vi "Enable or Disable Button.vi"(8 "Error In":errorcluster, 9 "Mark Selected Errors As Read Button Reference":refnum<vi>, 10 "MCL NewVal":i32[](array[numeric]), 11 "Handled Errors (MCL Display Order)":T1[](array[typedef])) -> (0 "Error Out":errorcluster)   [LabVIEW 2023, in "Error Manager.lvlib" / "Mark Selected Errors As Read Button.lvclass"]
doc: "This VI determines whether the \"Mark Selected Errors As Read\" button should be enabled or disabled and greyed out. The button should be enabled only when the user has selected one or more rows that represent unread errors.\n\nThis VI also controls the Boolean Text of the button. If 0 or 1 MCL rows are selected, the boolean text is set to \"Mark Selected Error As Read\". If two or more rows are selected, the boolean text is set to \"Mark Selected Errors As Read\"."
uses:
  Mark Selected Errors As Read Button.lvclass
  Mark Selected Errors As Read Button.lvclass/Mark Selected Errors As Read Button.ctl
  Private VIs/Read-Unread Status (enum).ctl
  Error Manager.lvlib
  Private VIs/Handled Error (cluster).ctl
panel:
  out "Number of MCL rows selected":i32
  # "Development\nControls or indicators that are useful for development or testing, but which are not outputs of the VI."
  # "Input\nInputs to the VI"
  # "Output\nOutputs of the VI"
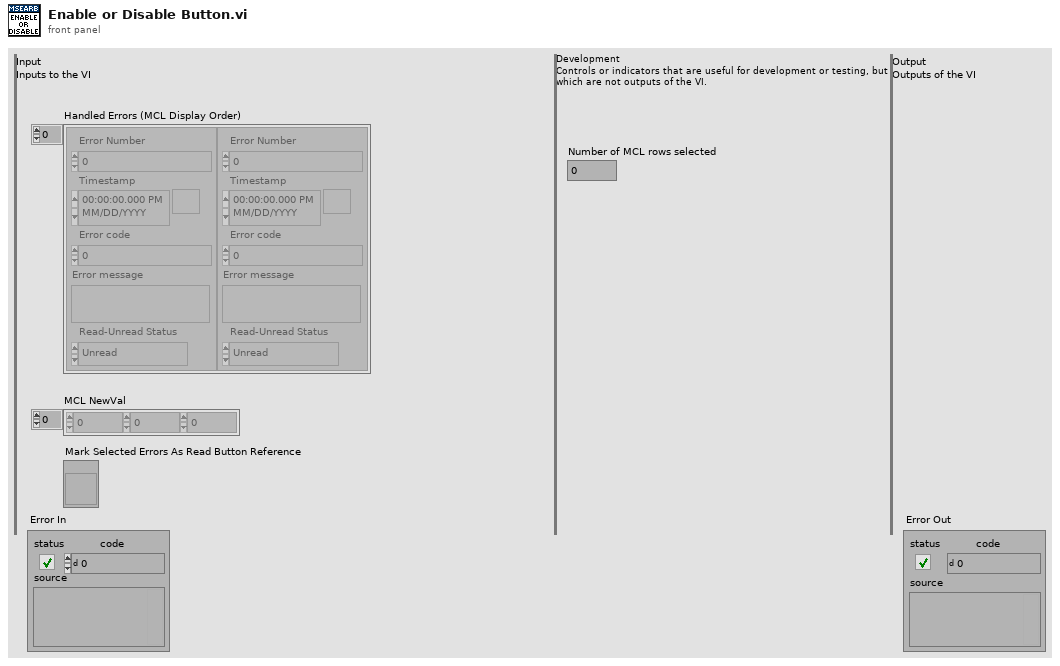
[diagram p1: front panel]
types:
  T1 = typedef "Error Manager.lvlib/Handled Error (cluster).ctl" = cluster{"Error Number":i32, "Timestamp":timestamp, "Error code":i32, "Error message":string, "Read-Unread Status":T2}
  T2 = typedef "Error Manager.lvlib/Read-Unread Status (enum).ctl" = enum16{"Unread", "Read"}
  T3 = enum8{"Enabled", "Disabled", "Disabled and Grayed Out"}
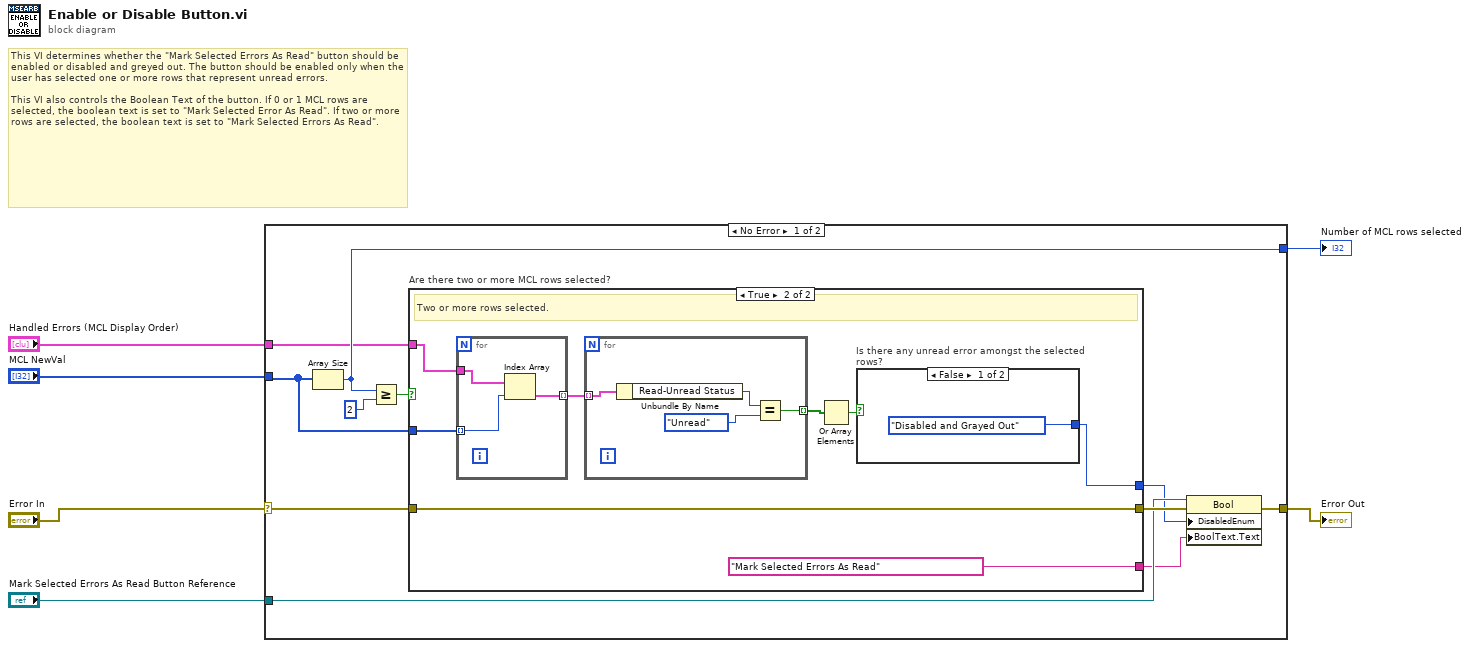
[diagram p0: block diagram]
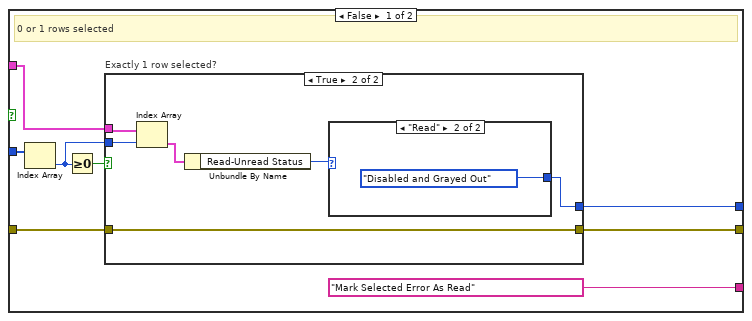
[diagram p2: hidden frame]
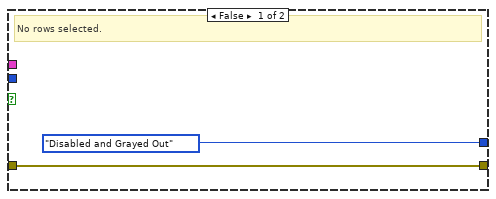
[diagram p3: hidden frame]
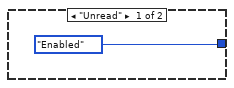
[diagram p4: hidden frame]
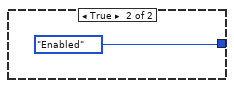
[diagram p5: hidden frame]
diagram:
  # "This VI determines whether the \"Mark Selected Errors As Read\" button should be enabled or disabled and greyed out. The button should be enabled only when the user has selected one or more rows that represent unread errors.\n\nThis VI also controls the Boolean Text of the button. If 0 or 1 MCL rows are selected, the boolean text is set to \"Mark Selected Error As Read\". If two or more rows are selected, the boolean text is set to \"Mark Selected Errors As Read\"."
  n1 = case shown="No Error" "Error In" {
    selector: "Error In" -> [w17 w53]
    tunnel: [w11 w53] -> w5
    tunnel: "Handled Errors (MCL Display Order)" -> [w8 _]
    tunnel: "MCL NewVal" -> [w12 _]
    tunnel: [w13 _] -> w2
    tunnel: "Mark Selected Errors As Read Button Reference" -> [w10 _]
    frame No Error {
      n2 = Array Size(array=w12) -> (size(s)=w13:i32)
      n3 = Greater Or Equal?(x=w13, y=2) -> (x >= y?=w14:bool)
      n4 = case "Are there two or more MCL rows selected?" shown="True" w14 {
        tunnel: w17 -> [w25 w43]
        tunnel: [w23 w43] -> w15
        tunnel: w12 -> [w24 w40]
        tunnel: [w21 w36] -> w9
        tunnel: w8 -> [w20 w41]
        tunnel: ["Mark Selected Error As Read" ("Boolean Text.Text") "Mark Selected Errors As Read" ("Boolean Text.Text")] -> w7
        frame False {
          # "0 or 1 rows selected"
          n5 = Index Array(array=w24) -> (element=w19:i32)  [unwired: 1 in]
          n6 = Greater Or Equal To 0?(x=w19) -> (x >= 0?=w22:bool)
          n7 = case "Exactly 1 row selected?" shown="True" w22 {
            tunnel: w25 -> [w27 w33]
            tunnel: [w27 w33] -> w23
            tunnel: [T3."Disabled and Grayed Out" ("Disabled") w28] -> w21
            tunnel: w20 -> [_ w31]
            tunnel: w19 -> [_ w32]
            frame False {
              # "No rows selected."
            }
            frame True {
              n8 = Index Array(array=w31, index=w32) -> (element=w30:T1)
              n9 = Unbundle By Name(w30) -> ("Read-Unread Status"=w29:T2)
              n10 = case shown="\"Read\"" w29 {
                tunnel: [T3."Enabled" ("Disabled") T3."Disabled and Grayed Out" ("Disabled")] -> w28
                frame "Unread" {
                }
                frame "Read" {
                }
              }
            }
          }
        }
        frame True {
          # "Two or more rows selected."
          n11 = for {
            tunnel: w41 -> [w52]
            tunnel: w40 -> [w51] mode=indexing
            tunnel: [w50] -> w39 mode=indexing
            n12 = Index Array(array=w52, index=w51) -> (element=w50:T1)
          }
          n13 = for {
            tunnel: w39 -> [w49] mode=indexing
            tunnel: [w46] -> w38 mode=indexing
            n14 = Unbundle By Name(w49) -> ("Read-Unread Status"=w48:T2)
            n15 = Equal?(x=w48, y=Read-Unread_Status_(enum)."Unread") -> (x = y?=w46:bool)
          }
          n16 = Or Array Elements(Boolean array=w38) -> (logical OR=w37:bool)
          n17 = case "Is there any unread error amongst the selected rows?" shown="False" w37 {
            tunnel: [T3."Disabled and Grayed Out" ("Disabled") T3."Enabled" ("Disabled")] -> w36
            frame False {
            }
            frame True {
            }
          }
        }
      }
      n18 = property class="Bool"(reference=w10, error in=w15, "DisabledEnum"=w9, "BoolText.Text"=w7) -> (error out=w11:errorcluster)  [unwired: 1 out]
    }
    frame Error {
    }
  }
  "Error Out" <- w5
  "Number of MCL rows selected" <- w2
